vi "MCL C Focus Set Focus Mode.vi"(10 "handle":i32, 11 "focusModeOn":bool) -> (3 "function return":i32)   [LabVIEW 2017, in "Madlib.lvlib"]
doc: "MADLIB_API int MCL_CFocusSetFocusMode(bool focusModeOn, int handle);"
uses:
  Madlib.lvlib
  Madlib.dll
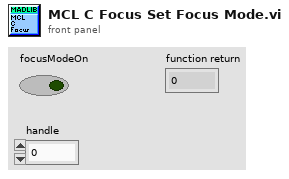
[diagram p1: front panel]
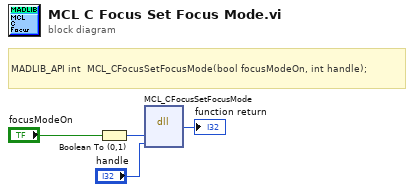
[diagram p0: block diagram]
diagram:
  # "MADLIB_API\tint\t\tMCL_CFocusSetFocusMode(bool focusModeOn, int handle);"
  n1 = Boolean To (0,1)(Boolean="focusModeOn") -> (0, 1=w2:i16)
  n2 = dll-call lib="C:/Users/francesco/dev/pump-probe/Piezo/lvlib/Madlib.*" fn="MCL_CFocusSetFocusMode"("focusModeOn"=w2, "handle"="handle") -> (→"function return":i32)  [unwired: 5 in, 2 out]
